vi "TelnetClient2.vi"(3 "Input Command":string="0 1.000 1 -1.0000 0 100 100", 4 "IP Address":string="192.168.1.128", 5 "Port #":i32=23) -> (0 "Telnet error":errorcluster, 1 "Transfer Command":string, 2 "Open Connection":string)   [LabVIEW 2013]
doc: "The Telnet Line Client VI uses the Telnet VIs to simulate a simple Telnet Window."
uses:
  <vilib>/addons/internet/NI_InternetTK_Core_VIs.lvlib
panel:
  # "Netburner Telnet Test Routine"
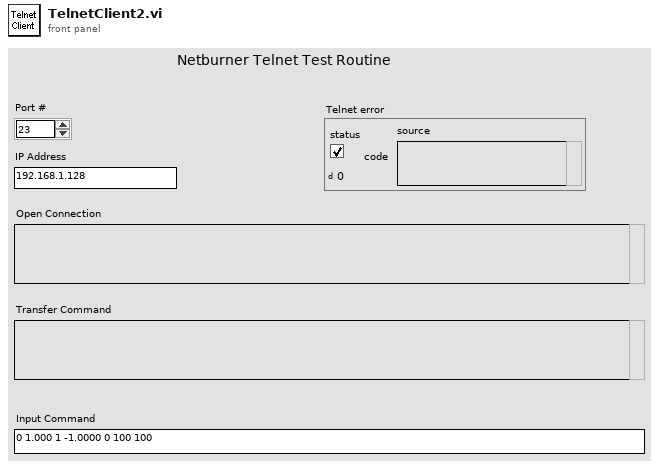
[diagram p1: front panel]
types:
  T1 = typedef "Telnet Session.ctl" = refnum<k1>
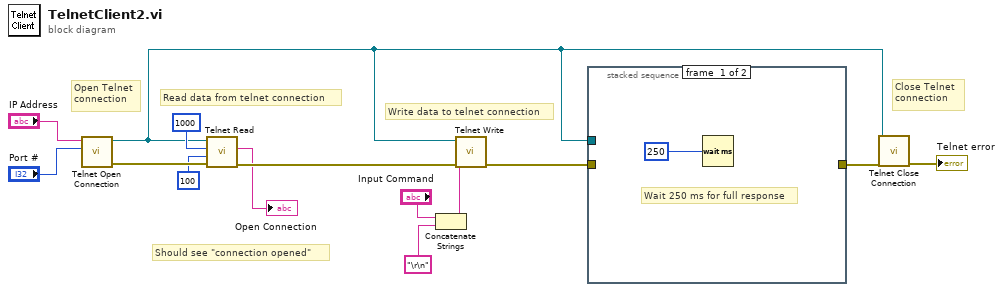
[diagram p0: block diagram]
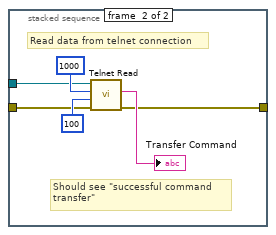
[diagram p2: hidden frame]
diagram:
  # "Should see \"connection opened\""
  # "Write data to telnet connection"
  # "Read data from telnet connection"
  # "Close Telnet \nconnection"
  # "Open Telnet\nconnection"
  n1 = call <vilib>:"Telnet Open Connection.vi"("remote port (23)"="Port #", "address"="IP Address") -> ("error out"=w12:errorcluster, "telnet connection"=w2:T1)  [unwired: 2 in, 6 out]
  n2 = call <vilib>:"Telnet Read.vi"("error in (no error)"=w12, "timeout ms (25000)"=100, "bytes to read"=1000, "telnet connection"=w2) -> ("error out"=w6:errorcluster, "data out"=→"Open Connection":string)  [unwired: 4 out]
  n3 = Concatenate Strings("Input Command", "\r\n") -> (w7:string)
  n4 = call <vilib>:"Telnet Write.vi"("error in (no error)"=w6, "data in"=w7, "telnet connection"=w2) -> ("error out"=w5:errorcluster)  [unwired: 1 in, 5 out]
  n5 = stacked-sequence {
    tunnel: w5 -> [_ w19]
    tunnel: w2 -> [_ w17]
    tunnel: [_ w16] -> w1
    frame #0 {
      # "Wait 250 ms for full response"
      n6 = Wait (ms)(milliseconds to wait=250) -> ()  [unwired: 1 out]
    }
    frame #1 {
      # "Should see \"successful command\ntransfer\""
      # "Read data from telnet connection"
      n7 = call <vilib>:"Telnet Read.vi"("error in (no error)"=w19, "timeout ms (25000)"=100, "bytes to read"=1000, "telnet connection"=w17) -> ("error out"=w16:errorcluster, "data out"=→"Transfer Command":string)  [unwired: 4 out]
    }
  }
  n8 = call <vilib>:"Telnet Close Connection.vi"("error in (no error)"=w1, "telnet connection"=w2) -> ("error out"=→"Telnet error":errorcluster)  [unwired: 9 out]
